vi "Initialize Session.vi"(8 "error in (no error)":errorcluster, 9 "Initialize_Info":T1, 10 "session reservation":refnum<class "Session Reservation.lvclass">, 11 "KeysightDMM in":refnum<class "KeysightDmm.lvclass">) -> (0 "error out":errorcluster, 3 "KeysightDMM out":refnum<class "KeysightDmm.lvclass">)   [LabVIEW 2021, in "KeysightDmm.lvclass"]
uses:
  KeysightDmm.lvclass
  C:/Program Files/National Instruments/LabVIEW 2021/vi.lib/Plug-In SDKs/Sessions/Instrument/ISession Factory/ISession Factory.lvclass
  Abstract_Instrument/TypeDef/Initialize_Info.ctl
  <vilib>/Plug-In SDKs/Clients/Session Management V1/Session Reservation/Initialize and Close Session Behavior.ctl
  <vilib>/Plug-In SDKs/Clients/Session Management V1/Session Reservation/Session Reservation.lvclass
  KeysightDmm.lvclass/KeysightDmm.ctl
  b5e2807c-68dc-4833-bbf3-7dc6427d04ea.vi
  <vilib>/Plug-In SDKs/Clients/Session Management V1/Session Reservation/Initialize Sessions with Retry.vi
  Abstract_Instrument/Abstract_Instrument.lvclass
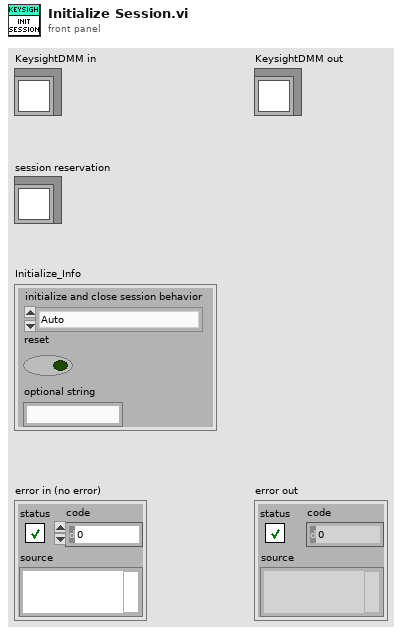
[diagram p1: front panel]
types:
  T1 = typedef "Abstract_Instrument.lvclass/Initialize_Info.ctl" = cluster{"initialize and close session behavior":T2, "reset":bool, "optional string":string}
  T2 = typedef "NI Session Management V1 Client.lvlib/Session Reservation.lvclass/Initialize and Close Session Behavior.ctl" = enum16{"Auto", "Initialize and Close", "Attach and Detach", "Initialize and Detach", "Attach and Close"}
  T3 = cluster{"Baud Rate":u32, "Parity":u16, "Data Bits":u16}
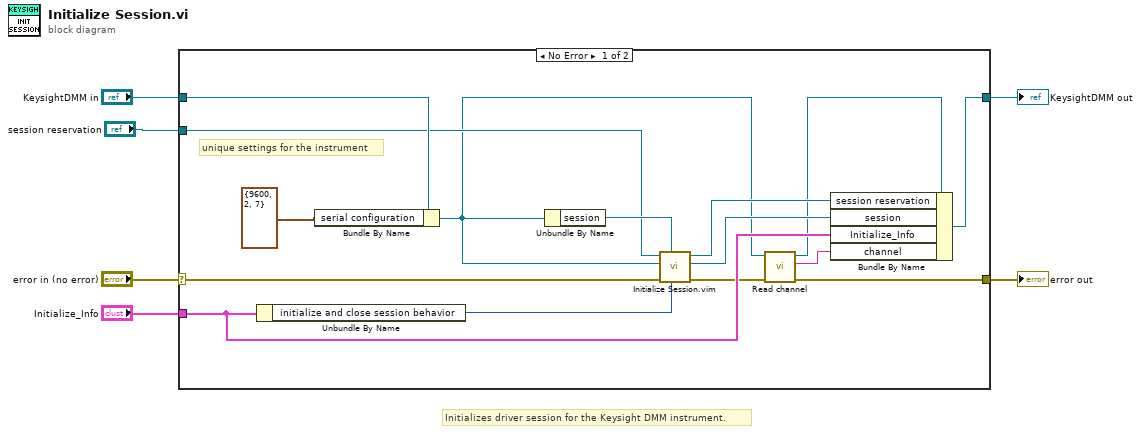
[diagram p0: block diagram]
diagram:
  # "Initializes driver session for the Keysight DMM instrument."
  n1 = case shown="No Error" "error in (no error)" {
    selector: "error in (no error)" -> [w19 w22]
    tunnel: [w10 w22] -> w3
    tunnel: [w18 w23] -> w2
    tunnel: "KeysightDMM in" -> [w17 w23]
    tunnel: "session reservation" -> [w15 _]
    tunnel: "Initialize_Info" -> [w12 _]
    frame No Error {
      # "unique settings for the instrument"
      n2 = Unbundle By Name(w12) -> ("initialize and close session behavior"=w14:T2)
      n3 = Bundle By Name(cluster=w17, "serial configuration"=T3 {"Baud Rate"=9600, "Parity"=2, "Data Bits"=7}) -> (w9:refnum<class "KeysightDmm.lvclass">)
      n4 = Unbundle By Name(w9) -> ("session"=w16:refnum<visa-resource-name>)
      n5 = call "Initialize Session.vim"("initialize and close session behavior"=w14, "session type"=w16, "error in"=w19, "session factory"=w9, "session reservation in"=w15) -> ("error out"=w11:errorcluster, "session"=w20:refnum<visa-resource-name>, "session reservation out"=w13:refnum<class "Session Reservation.lvclass">)  [unwired: 3 in, 1 out]
      n6 = call-dynamic "Read channel.vi"("error in (no error)"=w11, "Abstract_Instrument in"=w9) -> ("error out"=w10:errorcluster, "channel"=w7:string, "Abstract_Instrument out"=w8:refnum<class "KeysightDmm.lvclass">)  [unwired: 7 in]
      n7 = Bundle By Name(cluster=w8, "session reservation"=w13, "session"=w20, "Initialize_Info"=w12, "channel"=w7) -> (w18:refnum<class "KeysightDmm.lvclass">)
    }
    frame Error {
    }
  }
  "error out" <- w3
  "KeysightDMM out" <- w2
